vi "GLIMPSE Average fields.vi"(1 "Field buffer In":T1, 2 "Image in":T1) -> (0 "Field buffer Out":T1)   [LabVIEW 2011]
uses:
  <vilib>/vision/Image Controls.llb/IMAQ Image.ctl
  GLIMPSE Globals.vi
  <vilib>/vision/NI_Vision_Development_Module.lvlib
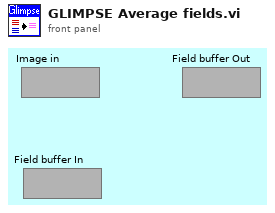
[diagram p1: front panel]
types:
  T1 = typedef "IMAQ Image.ctl" = refnum<image>
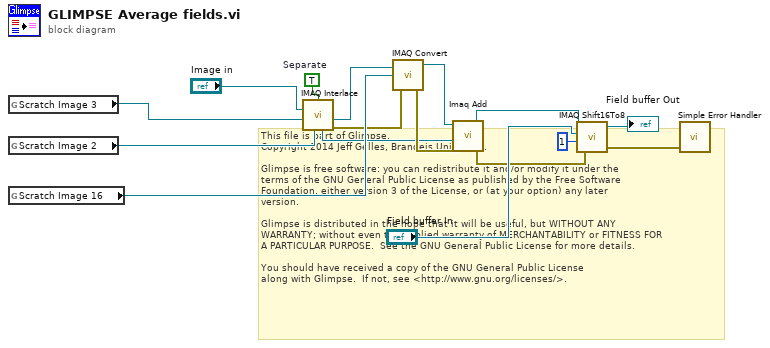
[diagram p0: block diagram]
diagram:
  w15 = TRUE  # Separate
  # "This file is part of Glimpse. \nCopyright 2014 Jeff Gelles, Brandeis University.    \n\nGlimpse is free software: you can redistribute it and/or modify it under the \nterms of the GNU General Public License as published by the Free Software \nFoundation, either version 3 of the License, or (at your option) any later \nversion.\n\nGlimpse is distributed in the hope that it will be useful, but WITHOUT ANY \nWARRANTY; without even the implied warranty of MERCHANTABILITY or FITNESS FOR \nA PARTICULAR PURPOSE.  See the GNU General Public License for more details.\n\nYou should have received a copy of the GNU General Public License\nalong with Glimpse.  If not, see <http://www.gnu.org/licenses/>."
  n1 = global read "GLIMPSE Globals.vi" "Scratch Image 3"() -> (w14:T1)
  n2 = global read "GLIMPSE Globals.vi" "Scratch Image 2"() -> (w13:T1)
  n3 = global read "GLIMPSE Globals.vi" "Scratch Image 16"() -> (w11:T1)
  n4 = call "IMAQ Interlace"("Image Even"=w14, "Image Odd"=w13, "Image Frame"="Image in", "Interlace/Separate (Interlace)"=w15) -> ("Image Odd Out"=w7:T1, "Image Even Out"=w12:T1, "error out"=w10:errorcluster)  [unwired: 1 in, 1 out]
  n5 = call "IMAQ Convert"("error in (no error)"=w10, "Image Dst"=w11, "Image Src"=w12) -> ("error out"=w9:errorcluster, "Image Dst Out"=w8:T1)  [unwired: 1 out]
  n6 = call "Imaq Add"("Image Src A"=w8, "Image Src B"=w7, "error in (no error)"=w9) -> ("Image Dst Out"=w5:T1, "error out"=w3:errorcluster)  [unwired: 2 in, 2 out]
  n7 = call "IMAQ Shift16To8"("error in (no error)"=w3, "Shift Value"=1, "Image Dst"="Field buffer In", "Image Src"=w5) -> ("error out"=w1:errorcluster, "Image Dst Out"=→"Field buffer Out":T1)  [unwired: 1 out]
  n8 = call <vilib>:"Simple Error Handler.vi"("error in (no error)"=w1) -> ()  [unwired: 1 in, 8 out]
